vi "set gain.vi"(8 "error in (no error)":errorcluster, 11 "Cascade in":refnum<class "Cascade.lvclass">) -> (0 "error out":errorcluster, 3 "Cascade out":refnum<class "Cascade.lvclass">)   [LabVIEW 2012, in "Cascade.lvclass"]
uses:
  Cascade.lvclass
  Cascade.lvclass/Cascade.ctl
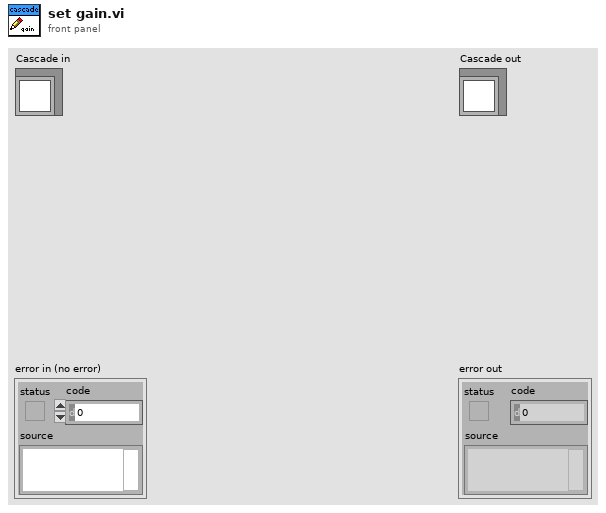
[diagram p1: front panel]
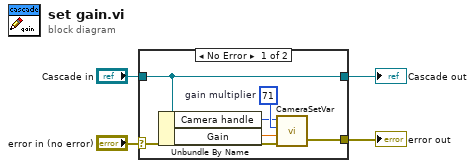
[diagram p0: block diagram]
diagram:
  n1 = case shown="No Error" "error in (no error)" {
    selector: "error in (no error)" -> [w6 w12]
    tunnel: [w9 w12] -> w3
    tunnel: [w10 w11] -> w1
    tunnel: "Cascade in" -> [w10 w11]
    frame No Error {
      w7 = u32 71  # gain multiplier
      n2 = Unbundle By Name(w10) -> ("Camera handle"=w5:u32, "Gain"=w8:dbl)
      n3 = call <userlib>:"CameraSetVar.vi"("error in"=w6, "Value"=w8, "Parameter ID"=w7, "Camera Handle"=w5) -> ("error out"=w9:errorcluster)  [unwired: 1 out]
    }
    frame Error {
    }
  }
  "error out" <- w3
  "Cascade out" <- w1
